vi "2020_day05.vi"() -> ()   [LabVIEW 2021]
uses:
  6eb49544-2da7-439a-8d24-4c096668e201.vi
  <vilib>/Comparison/Less/Less Functor/Less Functor.lvclass
panel:
  out "Task 2 - vacant seat":i32
  out "Task 1":i32
  in  "Switch":bool caption="Ex. Data  vs.  User Data"
  out "COL":i32
  out "ROW":i32
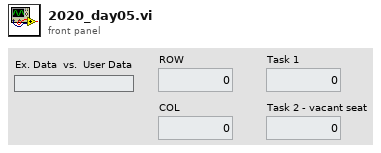
[diagram p1: front panel]
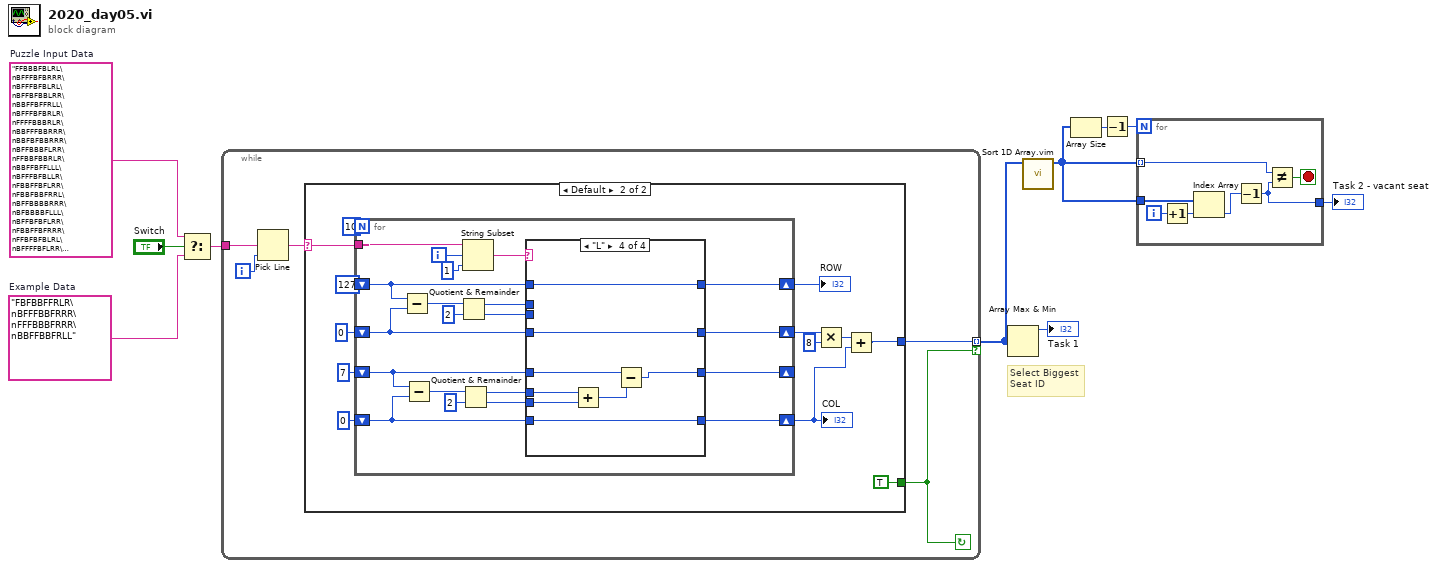
[diagram p0: block diagram]
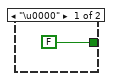
[diagram p2: hidden frame]
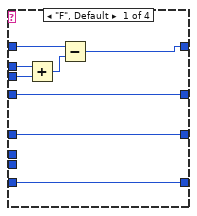
[diagram p3: hidden frame]
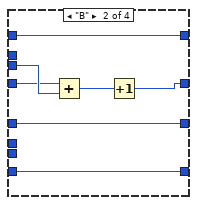
[diagram p4: hidden frame]
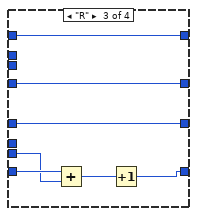
[diagram p5: hidden frame]
diagram:
  w10 = "FFBBBFBLRL\nBFFFBFBRRR\nBFFFBFBLRL\nBFFBFBBLRR\nBBFFBFFRLL\nBFFFBFBRLR\nFFFFBBBRLR\nBBFFFBBRRR\nBBFBFBBRRR\nBFFBBBFLRR\nFFBBFBBRLR\nBBFFBFFLLL\nBFFFBFBLLR\nFBBFFBFLRR\nFBBFBBFRRL\nBFFBBBBRRR\nBFBBBBFLLL\nBFFBFBFLRR\nFBBFFBFRRR\nFFBFBFBLRL\nBFFFFBFLRR\nFBBFFFFLRR\nBFFFBBBLLL\nBFBFFFBRLL\nFFBBBBBRLL\nFFBBFFBLLR\nFBFFBBFLRL\nFFBFFBBRRL\nBFBBBBFLLR\nBFFFFBFRRL\nBFFBFFFLLL\nFBFFFBFLRL\nFBBBFFFLLL\nFFBFBBFRLR\nFBBBFBFRRL\nBFBBBFBLLL\nFBFFFBFLRR\nFBFBFFBLRR\nBFFFFBFLRL\nFBFBFFFRRL\nFBBFBFBLRL\nFBBFFBFLLL\nFBFBBBBRRR\nFBBBBBFLRR\nFBBBFBBLLR\nFFFBFBFRLL\nFFFBBFFLRR\nBFBBFFBRRL\nFFBFBFBRRL\nFBFBBBBLRR\nBFFBBFFLLL\nFFFBFBBRRL\nBFBBFFFLRR\nFBFBFBFLRL\nBFBFFB..."  # Puzzle Input Data
  w9 = "FBFBBFFRLR\nBFFFBBFRRR\nFFFBBBFRRR\nBBFFBBFRLL"  # Example Data
  # "Select Biggest\nSeat ID"
  n1 = Select(t=w10, s="Switch", f=w9) -> (s? t:f=w7:string)
  n2 = while {
    tunnel: w7 -> [w11]
    tunnel: [w14] -> w6 mode=indexing if=w13
    i -> [w12]
    stop <- w13 continue-if-true
    n3 = Pick Line(multi-line string=w11, line index=w12) -> (output string=w15:string)  [unwired: 1 in]
    n4 = case shown="Default" w15 {
      selector: w15 -> [_ w19]
      tunnel: [FALSE TRUE] -> w13
      tunnel: [_ w17] -> w14
      frame "\u0000" {
      }
      frame Default {
        n5 = for {
          N: 10 -> [_]
          shift-right: [w39] -> w26
          shift-left: 127 -> [w44]
          tunnel: w19 -> [w48]
          shift-right: [w38] -> w23
          shift-left: 0 -> [w43]
          shift-right: [w36] -> _
          shift-left: 7 -> [w31]
          shift-right: [w37] -> w20
          shift-left: 0 -> [w32]
          i -> [w47]
          n6 = Subtract(x=w44, y=w43) -> (x-y=w42:i32)
          n7 = Subtract(x=w31, y=w32) -> (x-y=w33:i32)
          n8 = Quotient & Remainder(x=w42, y=2) -> (x-y*floor(x/y)=w40:i32, floor(x/y)=w41:i32)
          n9 = Quotient & Remainder(x=w33, y=2) -> (x-y*floor(x/y)=w35:i32, floor(x/y)=w34:i32)
          n10 = String Subset(string=w48, offset (0)=w47, length (rest)=1 ("length (rest)")) -> (substring=w45:string)
          n11 = case shown="\"L\"" w45 {
            tunnel: w41 -> [w57 w64 _ _]
            tunnel: w43 -> [w56 w62 w70 w78]
            tunnel: [w55 w63 w71 w79] -> w39
            tunnel: [w56 w60 w70 w78] -> w38
            tunnel: w44 -> [w54 w63 w71 w79]
            tunnel: w40 -> [w52 _ _ _]
            tunnel: w34 -> [_ _ w65 w76]
            tunnel: w32 -> [w50 w59 w67 w72]
            tunnel: [w51 w58 w66 w74] -> w36
            tunnel: [w50 w59 w69 w72] -> w37
            tunnel: w31 -> [w51 w58 w66 w77]
            tunnel: w35 -> [_ _ _ w75]
            frame "F", Default {
              n12 = Add(x=w52, y=w57) -> (x+y=w53:i32)
              n13 = Subtract(x=w54, y=w53) -> (x-y=w55:i32)
            }
            frame "B" {
              n14 = Add(x=w62, y=w64) -> (x+y=w61:i32)
              n15 = Increment(x=w61) -> (x+1=w60:i32)
            }
            frame "R" {
              n16 = Add(x=w67, y=w65) -> (x+y=w68:i32)
              n17 = Increment(x=w68) -> (x+1=w69:i32)
            }
            frame "L" {
              n18 = Add(x=w75, y=w76) -> (x+y=w73:i32)
              n19 = Subtract(x=w77, y=w73) -> (x-y=w74:i32)
            }
          }
        }
        "ROW" <- w26
        "COL" <- w20
        n20 = Multiply(x=w23, y=8) -> (x*y=w21:i32)
        n21 = Add(x=w21, y=w20) -> (x+y=w17:i32)
      }
    }
  }
  n22 = Array Max & Min(array=w6) -> (max value=→"Task 1":i32)  [unwired: 3 out]
  n23 = call "Sort 1D Array.vim"("unsorted array"=w6) -> ("sorted array"=w4:i32[])  [unwired: 10 in]
  n24 = Array Size(array=w4) -> (size(s)=w3:i32)
  n25 = Decrement(x=w3) -> (x-1=w2:i32)
  n26 = for {
    N: w2 -> [_]
    tunnel: w4 -> [w81] mode=indexing
    tunnel: w4 -> [w85]
    tunnel: [w80] -> w1
    i -> [w86]
    stop <- w83 stop-if-true
    n27 = Increment(x=w86) -> (x+1=w82:i32)
    n28 = Index Array(array=w85, index=w82) -> (element=w84:i32)
    n29 = Decrement(x=w84) -> (x-1=w80:i32)
    n30 = Not Equal?(x=w81, y=w80) -> (x != y?=w83:bool)
  }
  "Task 2 - vacant seat" <- w1
